vi "Calibration.vi"(6 "SN":T1, 7 "Show Front Panel":bool=TRUE, 8 "error in (no error)":errorcluster, 9 "file path (dialog if empty)":path=path "C:/Program Files/GE/Dryer Performance Test/CalibrationDates.txt", 10 "Calibration\nDue Date":T3 {"Chamber Temp" format="%<%x>T"; "Probe 2 Temp" format="%<%x>T"; "Probe 1 Temp" format="%<%x>T"; "TC Panel 2" format="%<%x>T"; "TC Panel 1" format="%<%x>T"; "NI DAQ Card 7" format="%<%x>T"; "NI DAQ Card 6" format="%<%x>T"; "NI DAQ Card 5" format="%<%x>T"; "NI DAQ Card 4" format="%<%x>T"; "NI DAQ Card 3" format="%<%x>T"; "NI DAQ Card 2" format="%<%x>T"; "NI DAQ Card 1" format="%<%x>T"; "Gas Meter Thermocouple" format="%<%x>T"; "Gas Meter Pressure Transducer" format="%<%x>T"; "Gas Meter" format="%<%x>T"; "Sentra Scale" format="%<%x>T"; "B-Tech Scale" format="%<%x>T"; "Barometer" format="%<%x>T"; "WT 500" format="%<%x>T"; "Chroma" format="%<%x>T"}, 11 "Calibration ID":T2) -> (0 "error out":errorcluster, 4 "OutputData":string[][](array[string]))   [LabVIEW 2012]
uses:
  Calibration.ctl
  CalibrationTime.ctl
  Calibration_SN.ctl
  <vilib>/Utility/file.llb/Write To Spreadsheet File (string).vi
panel:
  in  "Size":i32
  out "snta":string[](array[string])
  in  "Tab Control":enum32{"Calibration Dates", "File Location"}(tab)
  in  "Complete":bool
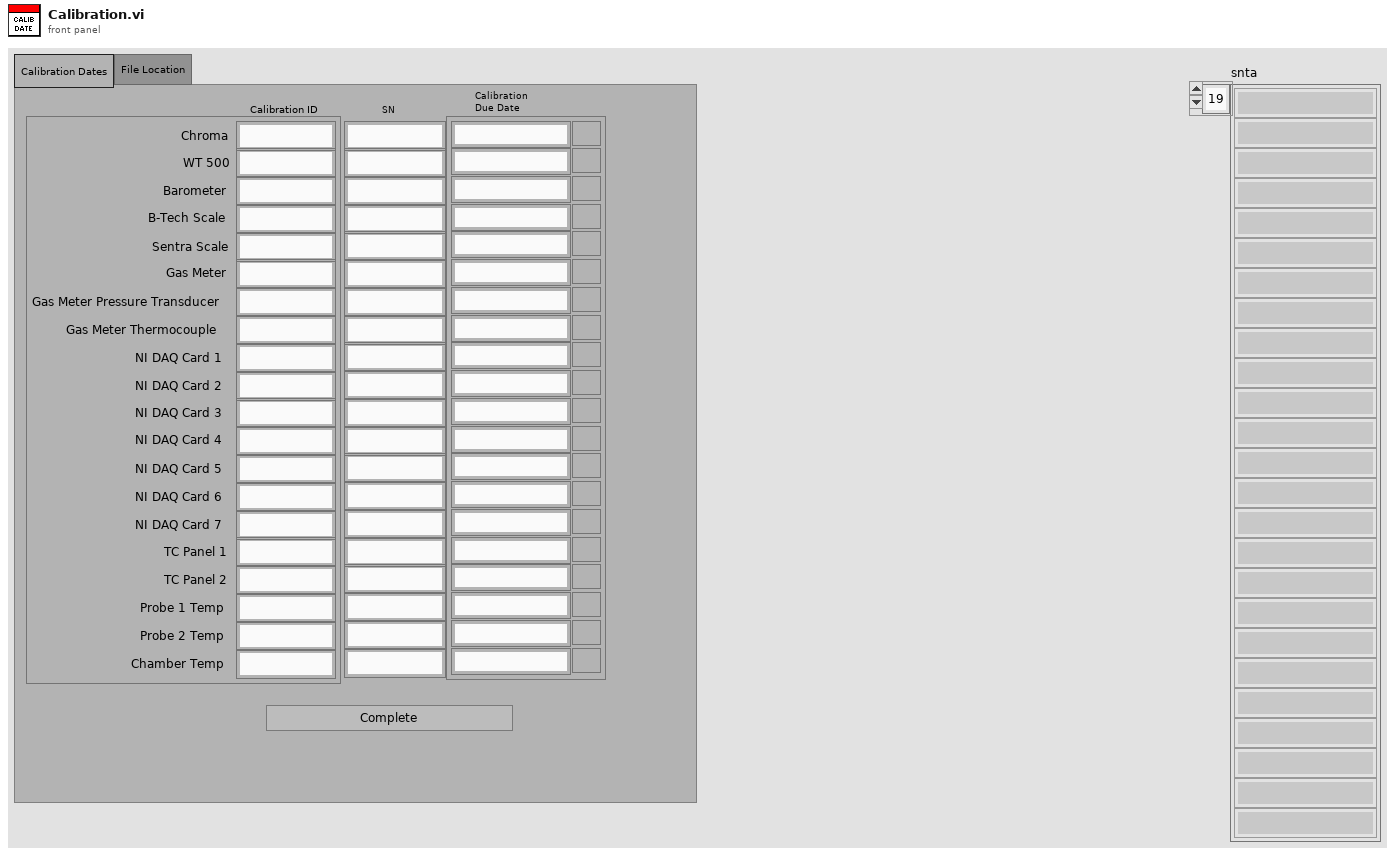
[diagram p1: front panel]
types:
  T1 = typedef "Calibration_SN.ctl" = cluster{"Chroma":string, "WT 500":string, "Barometer":string, "B-Tech Scale":string, "Sentra Scale":string, "Gas Meter":string, "Gas Meter Pressure Transducer":string, "Gas Meter Thermocouple":string, "NI DAQ Card 1":string, "NI DAQ Card 2":string, "NI DAQ Card 3":string, "NI DAQ Card 4":string, "NI DAQ Card 5":string, "NI DAQ Card 6":string, "NI DAQ Card 7":string, "TC Panel 1":string, "TC Panel 2":string, "Probe 1 Temp":string, "Probe 2 Temp":string, "Chamber Temp":string}
  T2 = typedef "Calibration.ctl" = cluster{"Chroma":string, "WT 500":string, "Barometer":string, "B-Tech Scale":string, "Sentra Scale":string, "Gas Meter":string, "Gas Meter Pressure Transducer":string, "Gas Meter Thermocouple":string, "NI DAQ Card 1":string, "NI DAQ Card 2":string, "NI DAQ Card 3":string, "NI DAQ Card 4":string, "NI DAQ Card 5":string, "NI DAQ Card 6":string, "NI DAQ Card 7":string, "TC Panel 1":string, "TC Panel 2":string, "Probe 1 Temp":string, "Probe 2 Temp":string, "Chamber Temp":string}
  T3 = typedef "CalibrationTime.ctl" = cluster{"Chroma":timestamp, "WT 500":timestamp, "Barometer":timestamp, "B-Tech Scale":timestamp, "Sentra Scale":timestamp, "Gas Meter":timestamp, "Gas Meter Pressure Transducer":timestamp, "Gas Meter Thermocouple":timestamp, "NI DAQ Card 1":timestamp, "NI DAQ Card 2":timestamp, "NI DAQ Card 3":timestamp, "NI DAQ Card 4":timestamp, "NI DAQ Card 5":timestamp, "NI DAQ Card 6":timestamp, "NI DAQ Card 7":timestamp, "TC Panel 1":timestamp, "TC Panel 2":timestamp, "Probe 1 Temp":timestamp, "Probe 2 Temp":timestamp, "Chamber Temp":timestamp}
  T4 = enum32{"invalid app kind", "Development System", "Run Time System", "Student Edition", "Embedded LabVIEW", "Evaluation", "Custom"}
  T5 = enum32{"Invalid", "Standard", "Closed", "Hidden", "Minimized", "Maximized"}
  T6 = cluster{"Core":cluster{"Current VI Reference":refnum<vi>, "Close Panel on Exit?":bool}, "Calibration\nDue Date":T3, "file path (dialog if empty)":path, "SN":T1, "Calibration ID":T2, "Total Array":string[][], "Size":i32}
  T7 = cluster{"Current VI Reference":refnum<vi>, "Close Panel on Exit?":bool}
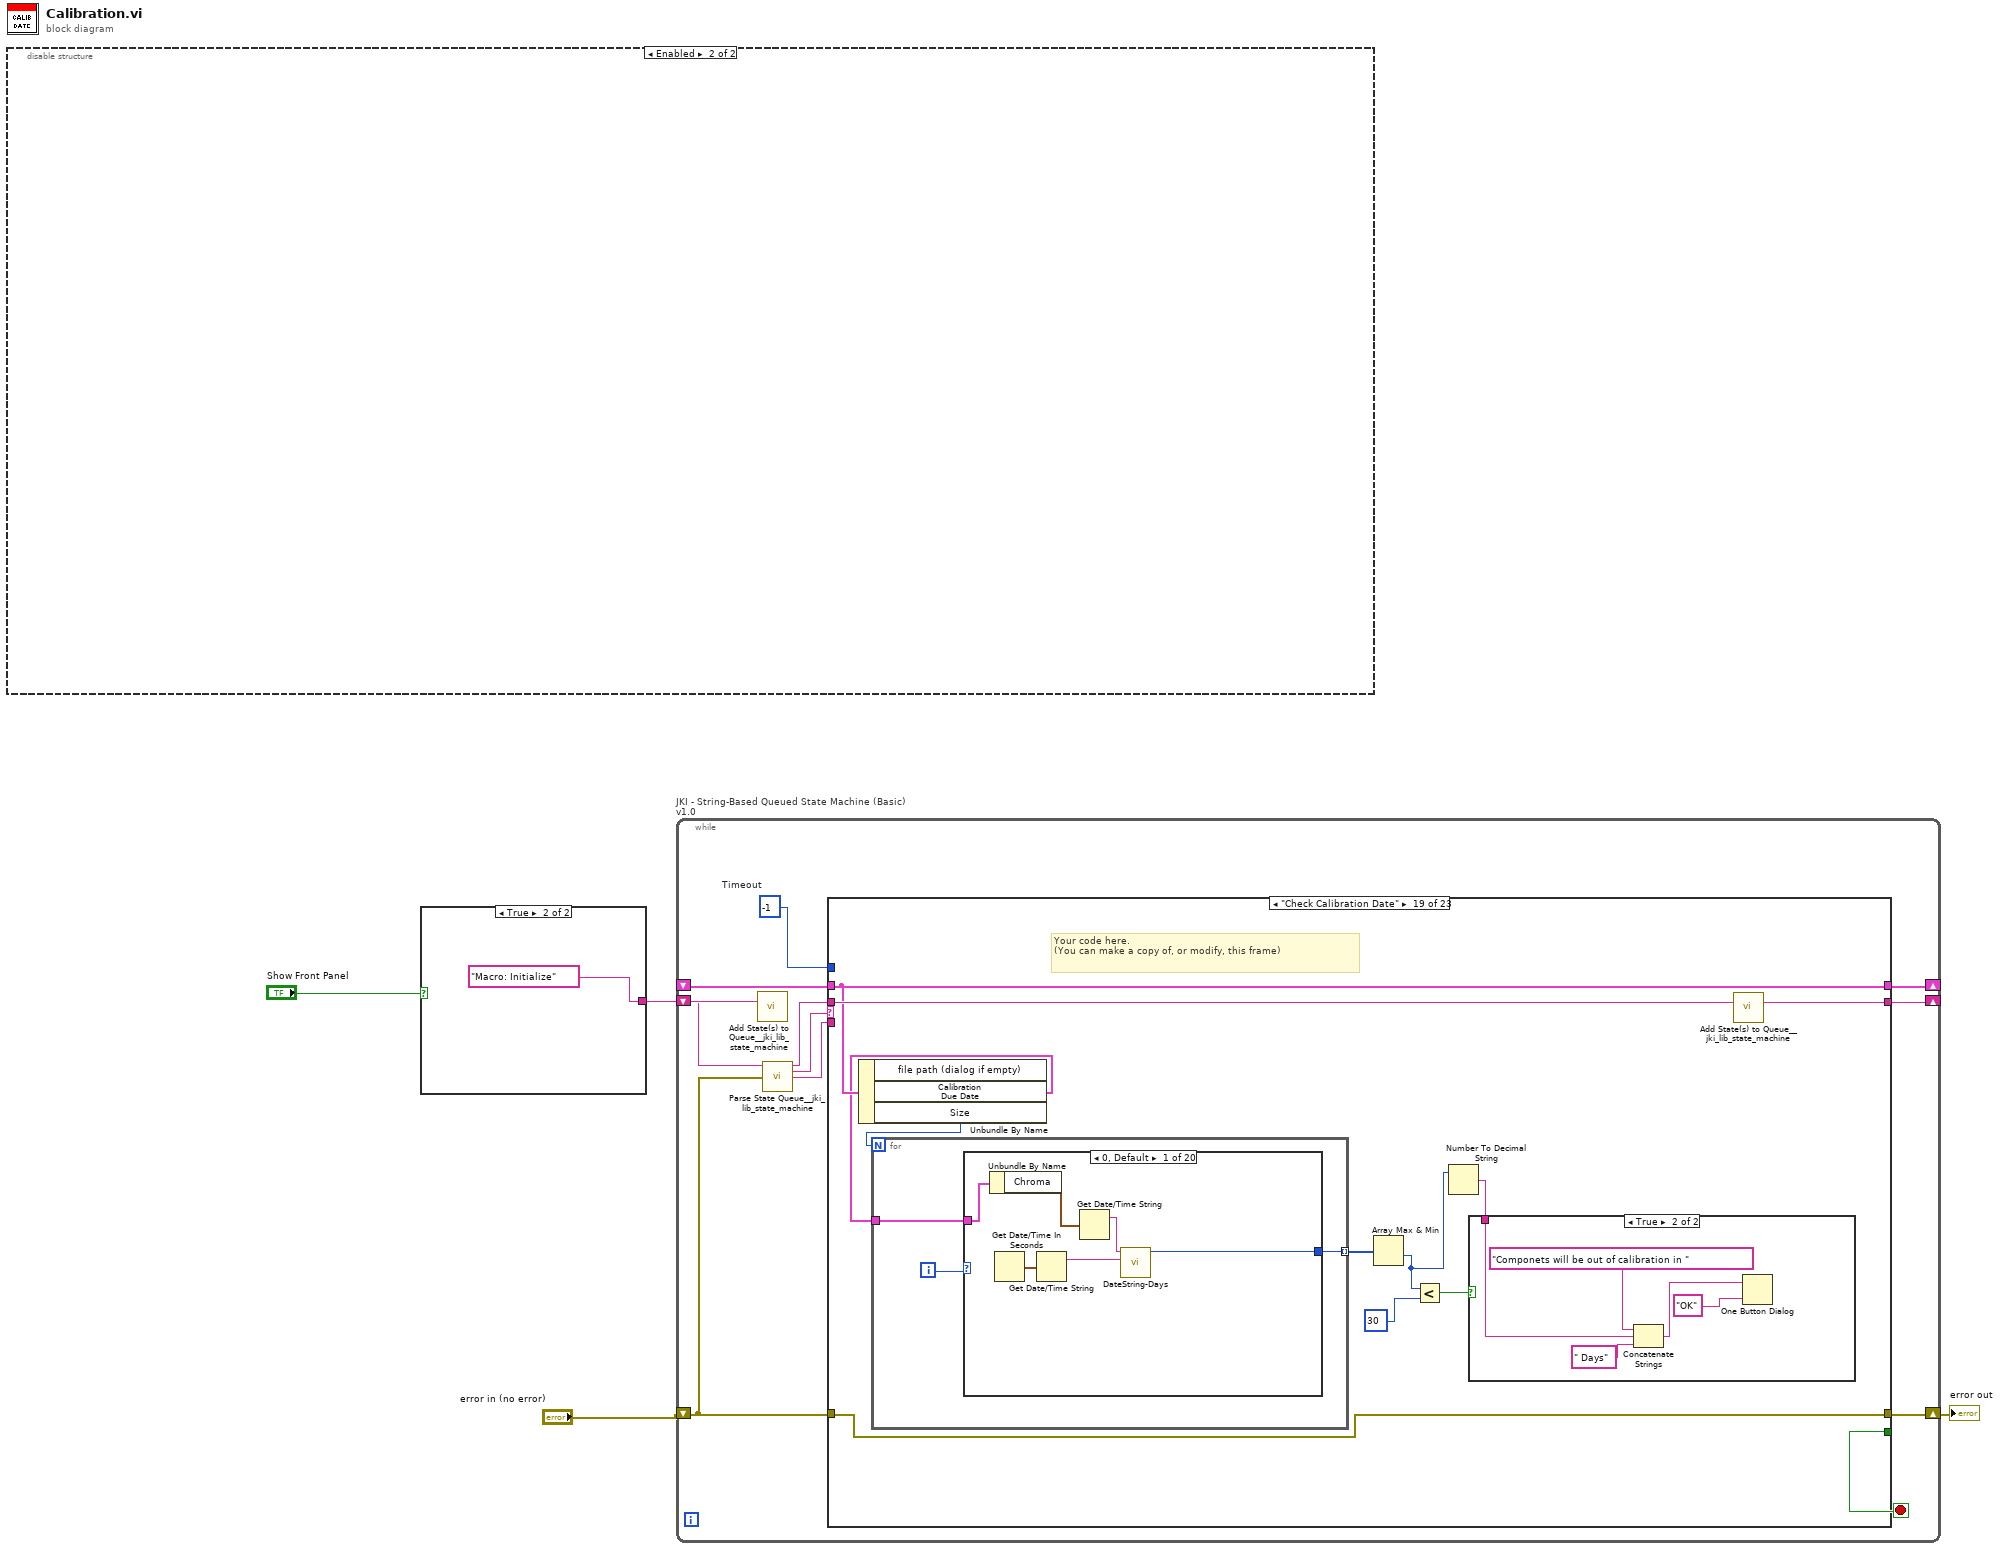
[diagram p0: block diagram]
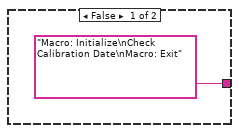
[diagram p2: hidden frame]
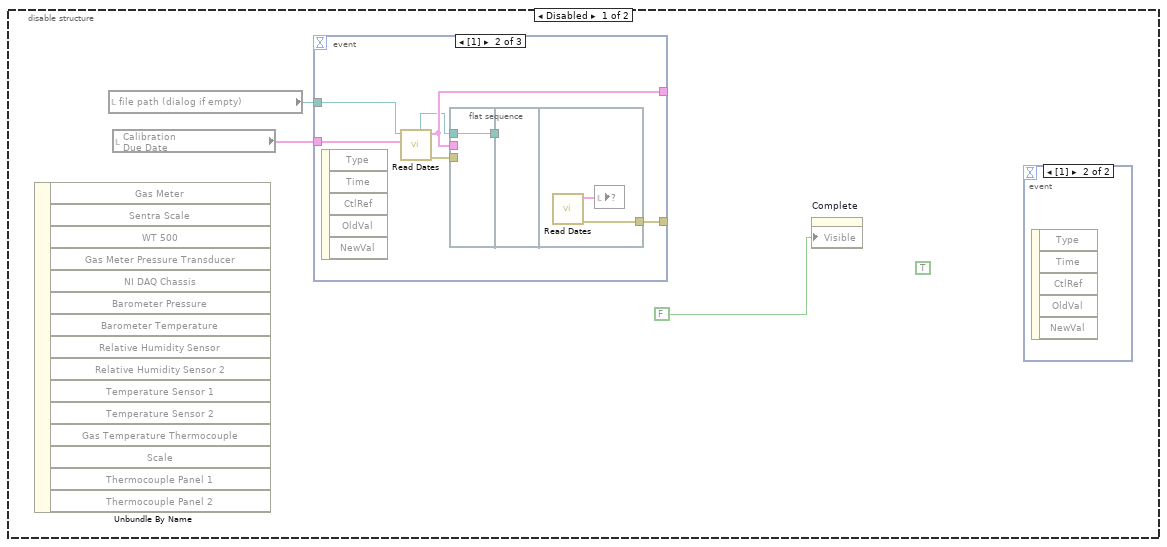
[diagram p3: hidden frame]
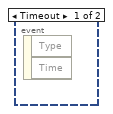
[diagram p4: hidden frame]
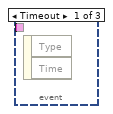
[diagram p5: hidden frame]
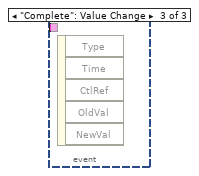
[diagram p6: hidden frame]
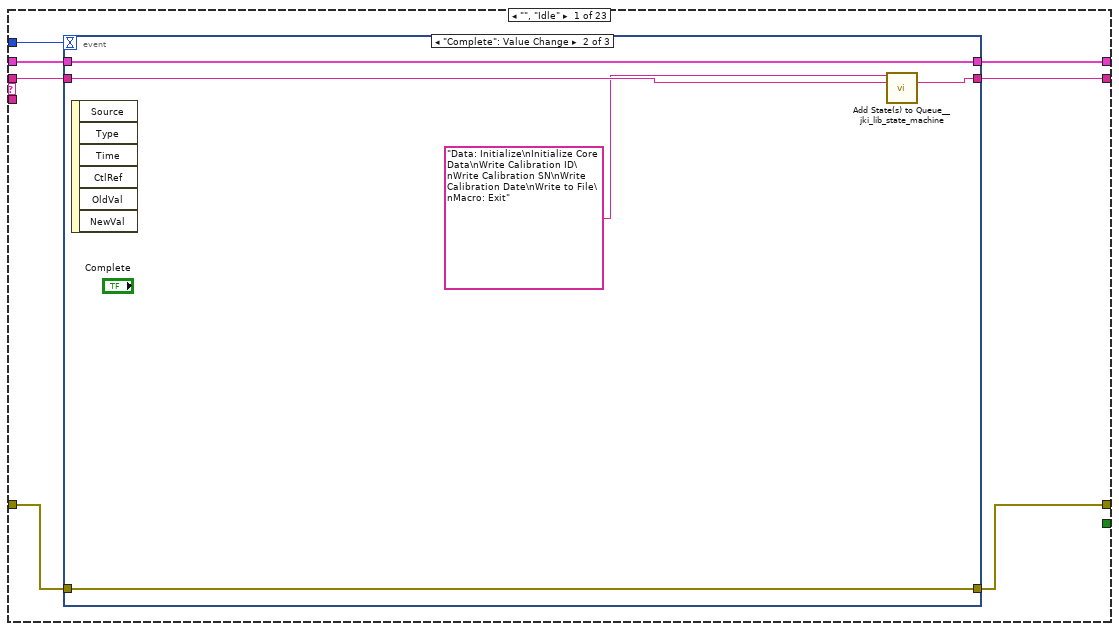
[diagram p7: hidden frame]
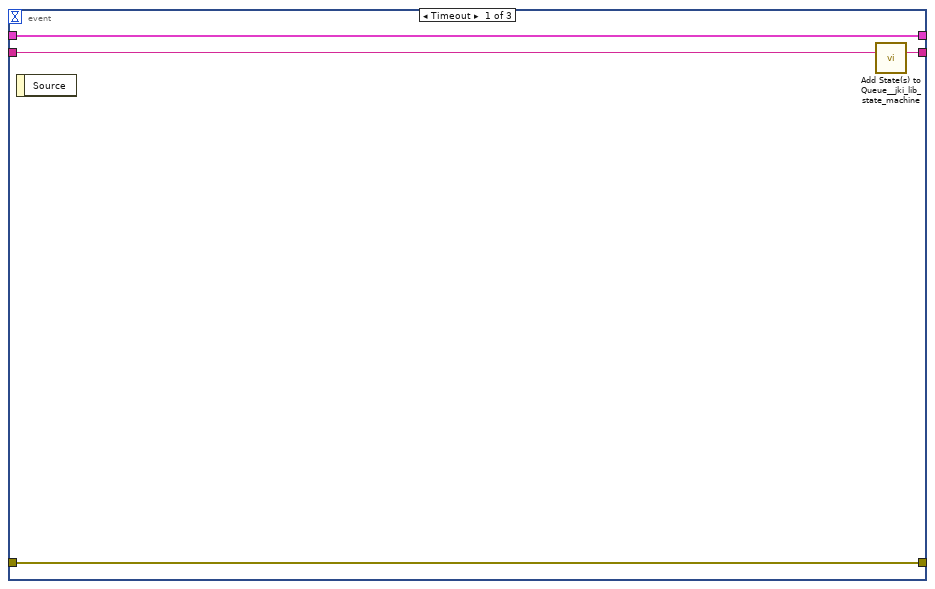
[diagram p8: hidden frame]
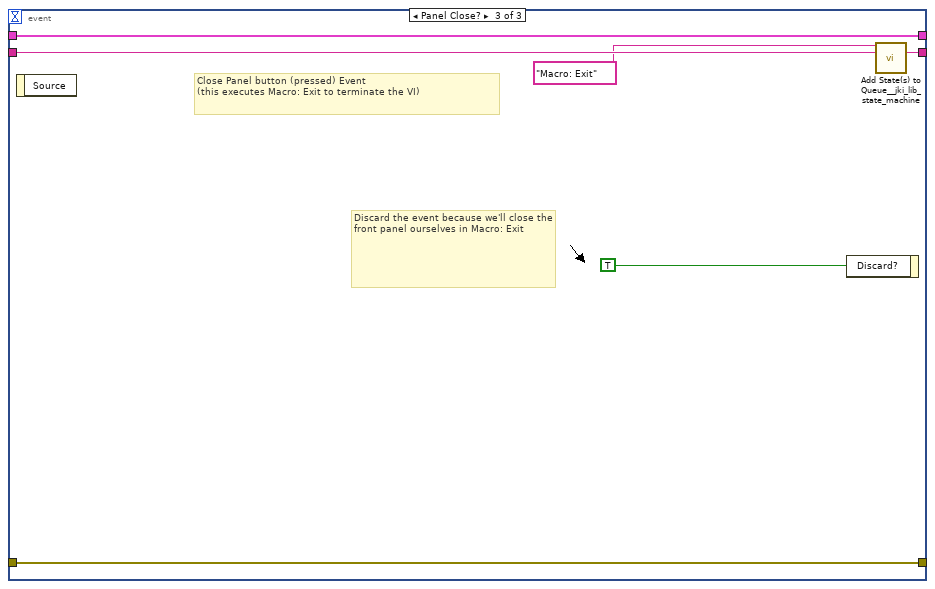
[diagram p9: hidden frame]
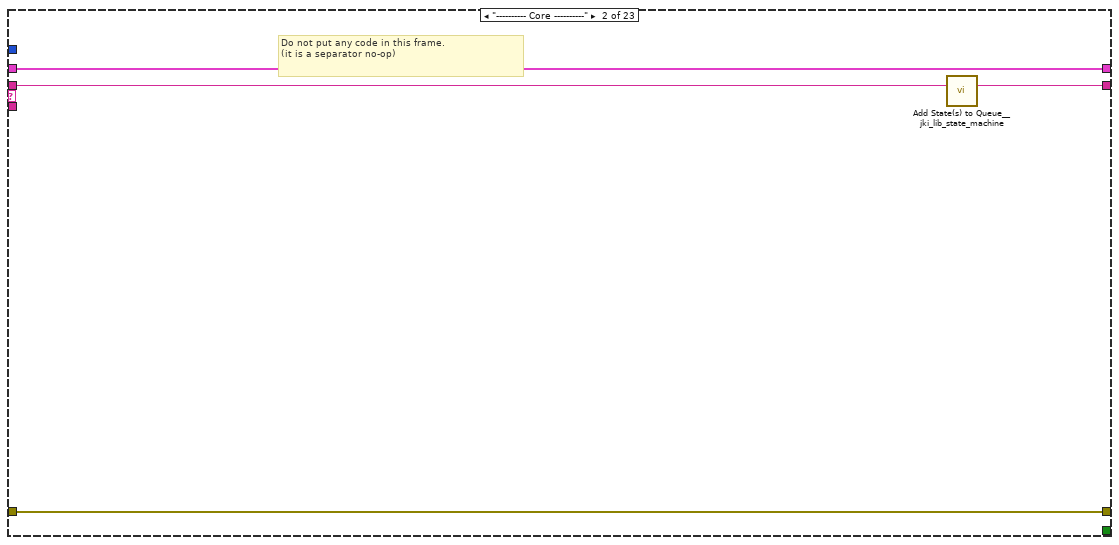
[diagram p10: hidden frame]
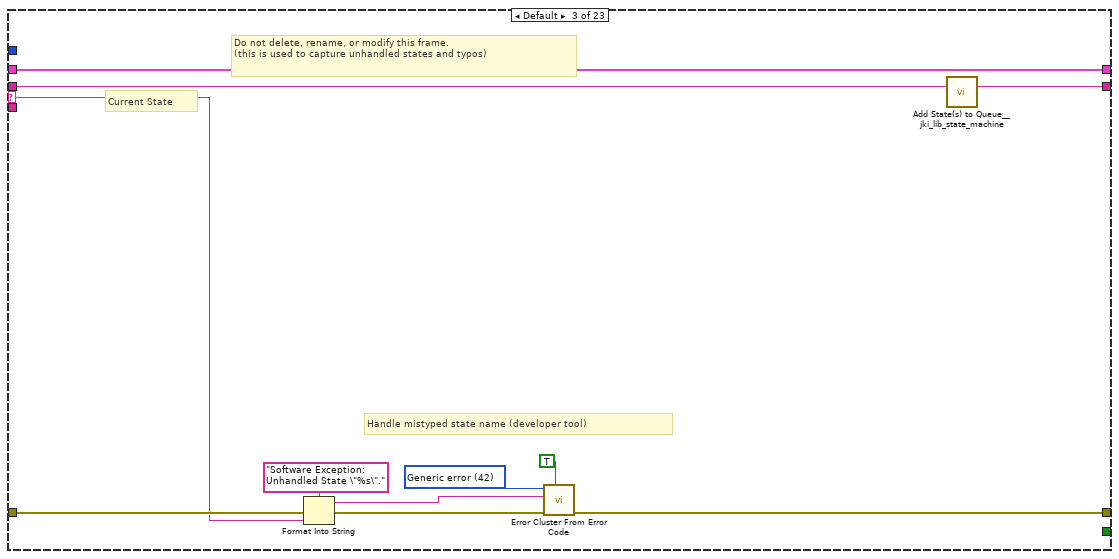
[diagram p11: hidden frame]
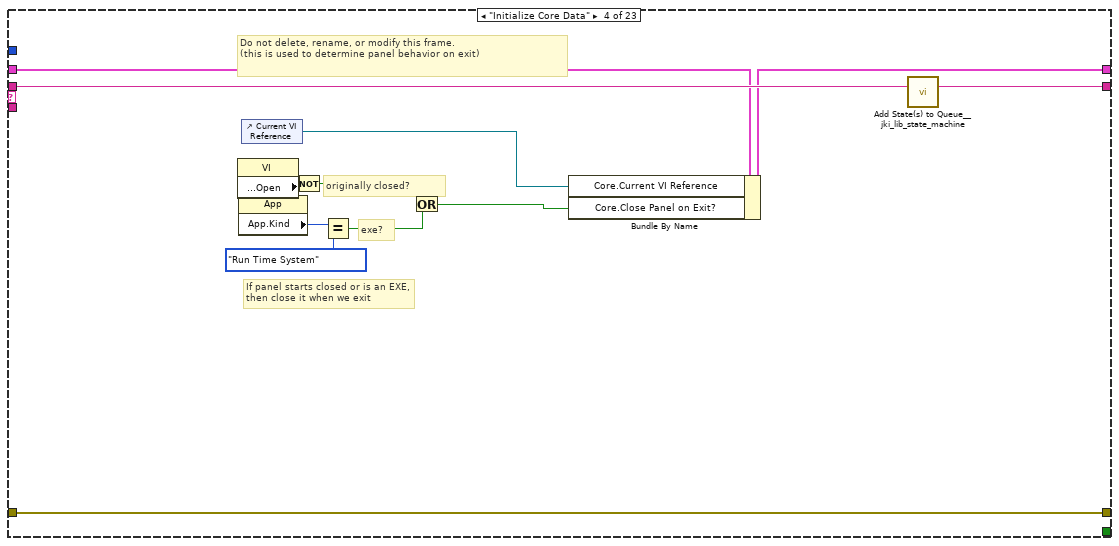
[diagram p12: hidden frame]
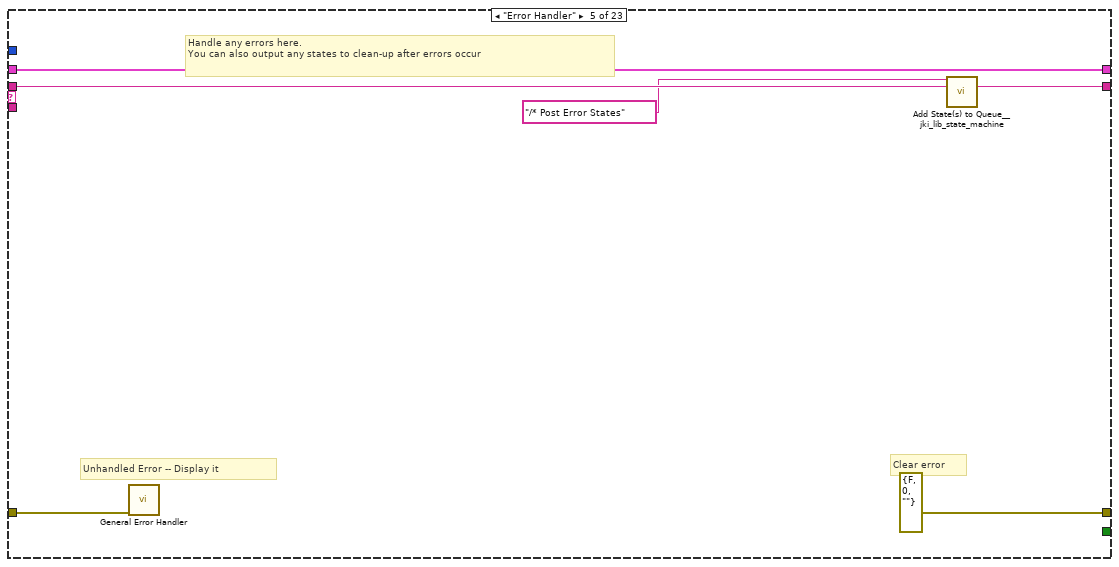
[diagram p13: hidden frame]
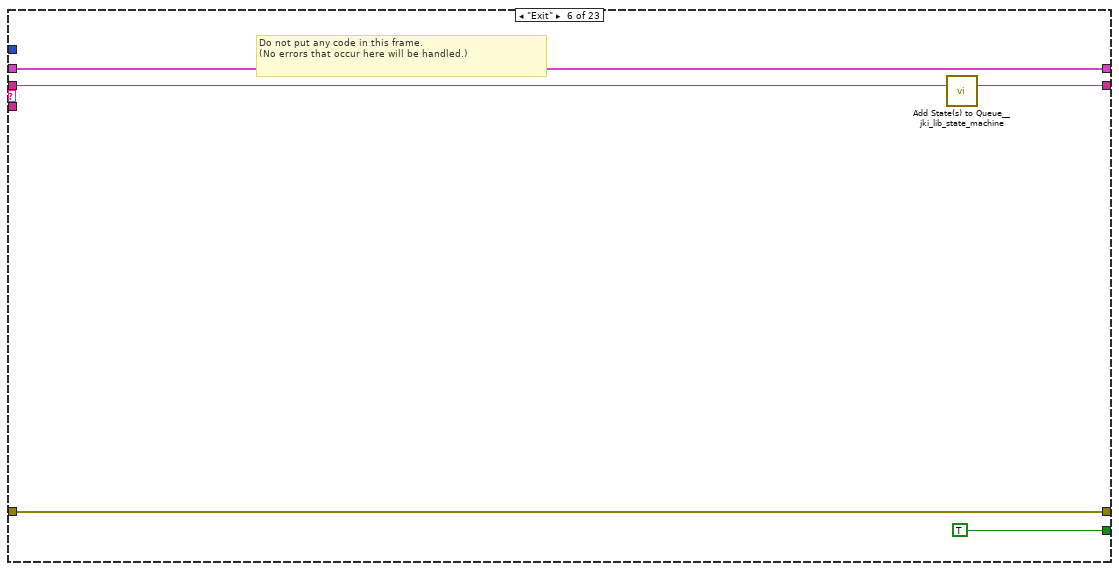
[diagram p14: hidden frame]
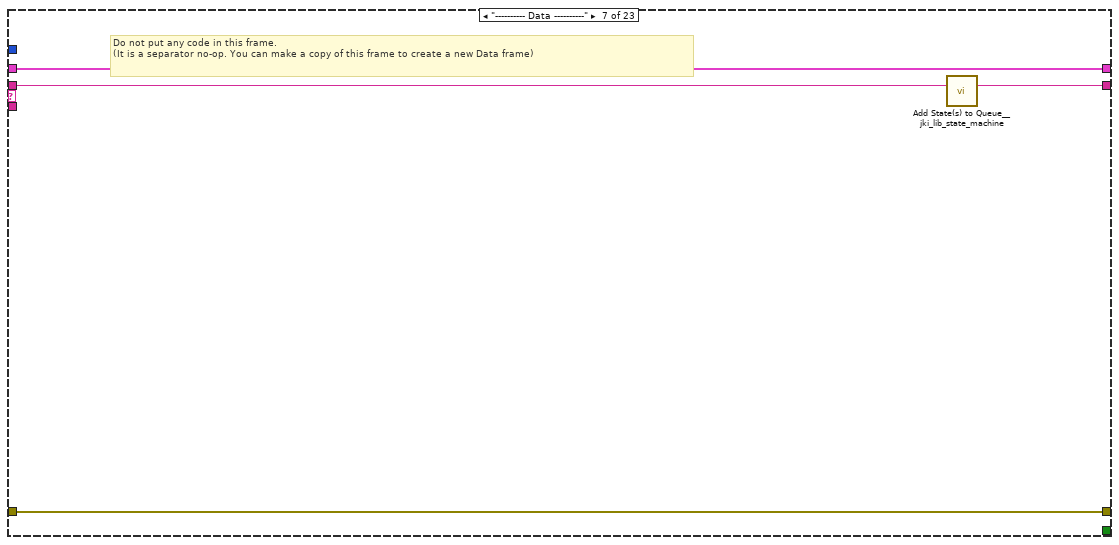
[diagram p15: hidden frame]
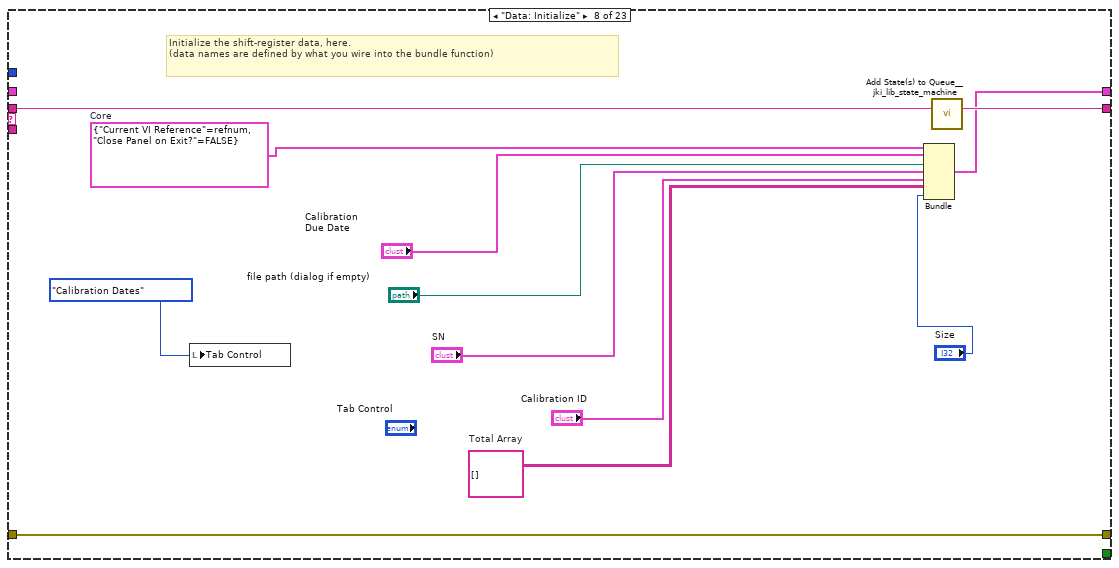
[diagram p16: hidden frame]
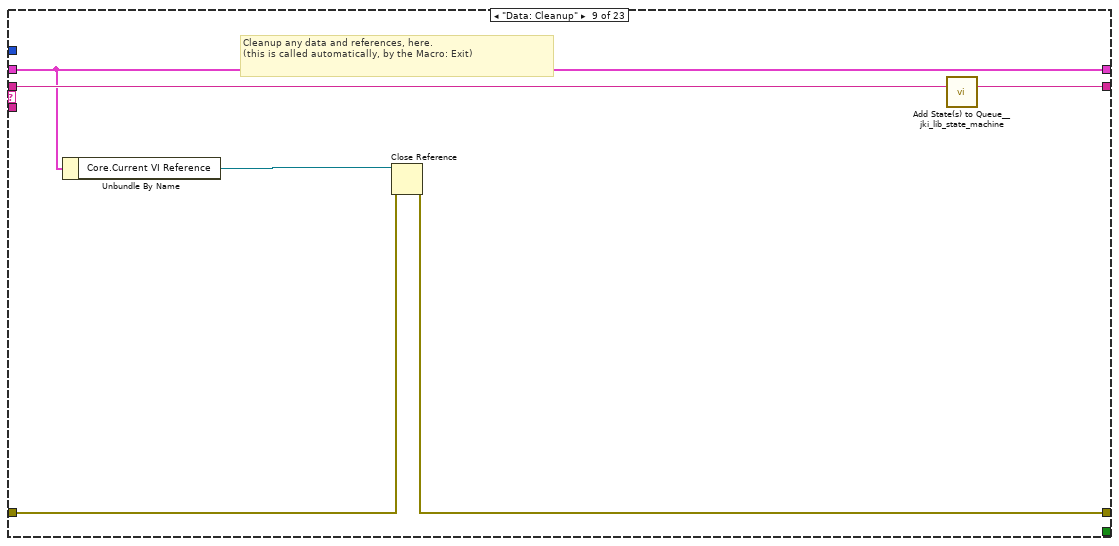
[diagram p17: hidden frame]
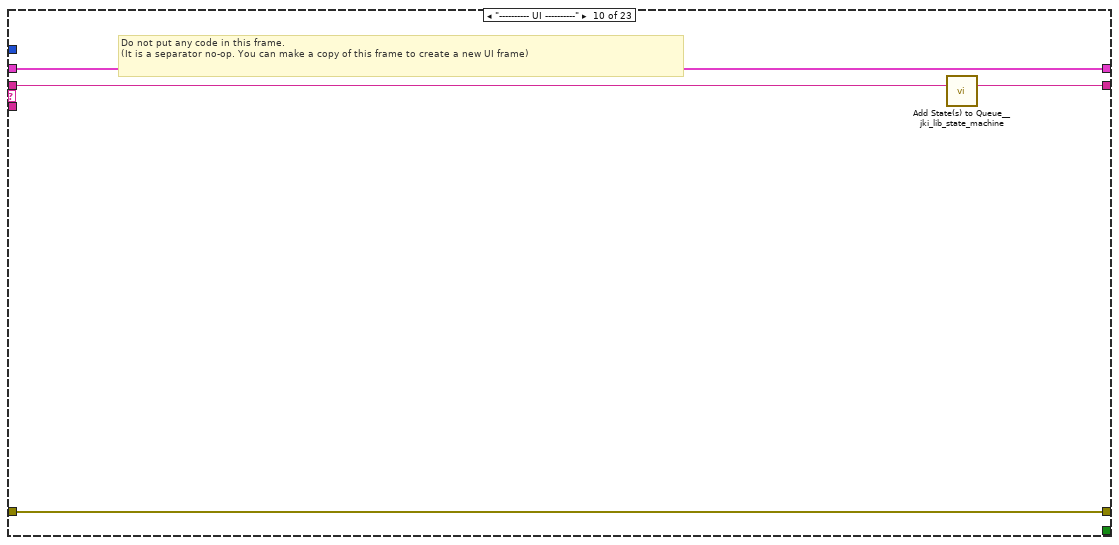
[diagram p18: hidden frame]
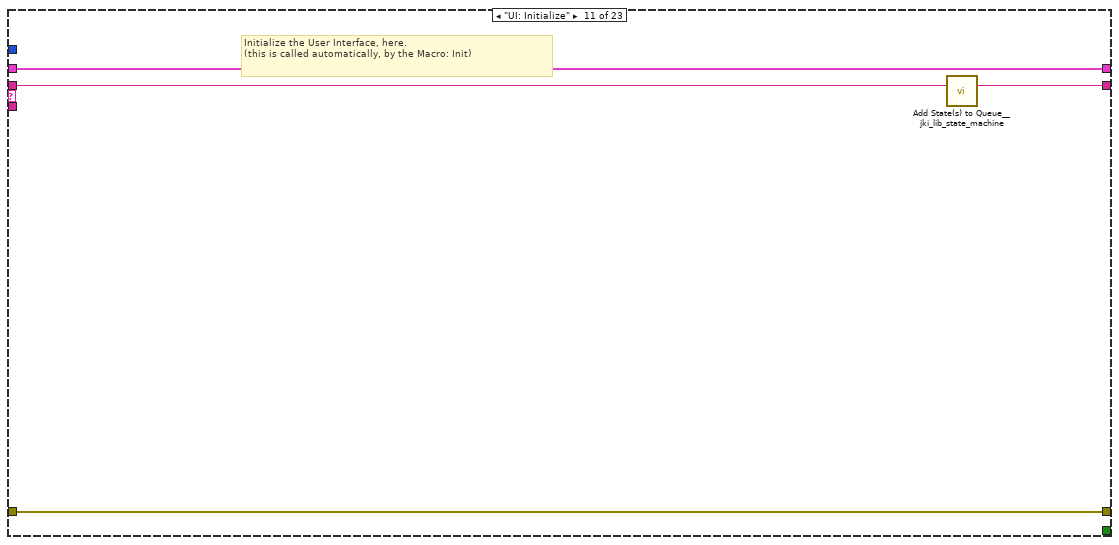
[diagram p19: hidden frame]
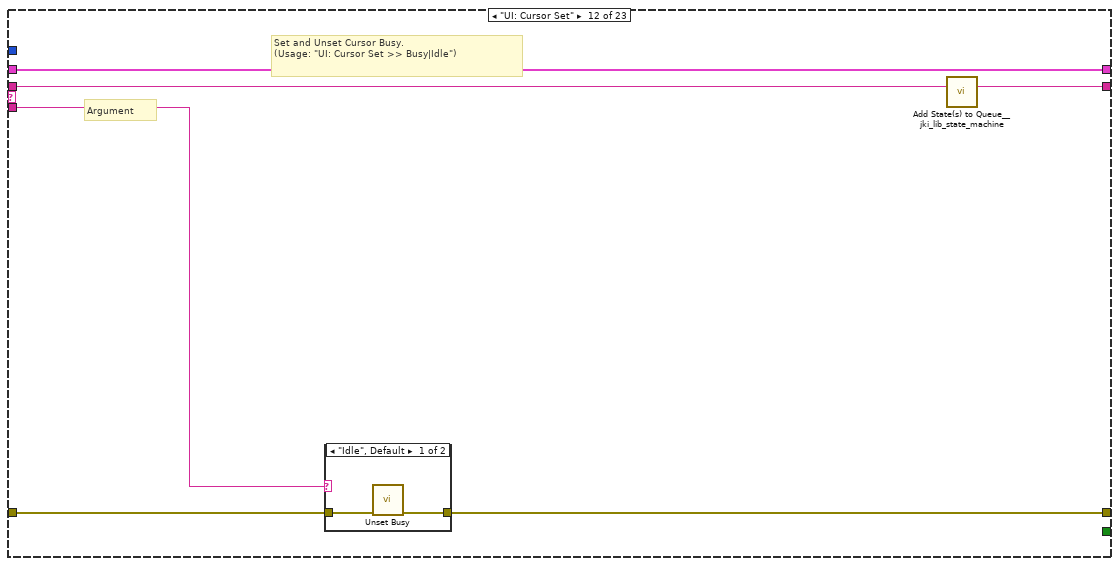
[diagram p20: hidden frame]
diagram:
  n1 = disable-structure shown="Enabled" {
    frame Disabled {
      w8 = TRUE ("Visible")
      n2 = Unbundle By Name() -> ()  [unwired: 1 in, 15 out]
      n3 = local read "file path (dialog if empty)"() -> (w6:path)
      n4 = local read "Calibration\nDue Date"() -> (w7:T3)
      n5 = event shown="[1]" {
        selector: _ -> [_ _ _]
        dyn-events: _ -> [_ _ _]
        timeout: _ -> [_ _ _]
        tunnel: [_ w13 _] -> _
        tunnel: [_ w17 _] -> _
        tunnel: w7 -> [_ w15 _]
        tunnel: w6 -> [_ w14 _]
        event Timeout {
          n6 = event-data() -> ()  [unwired: 1 in, 2 out]
        }
        event #1 (no event record) {
          n7 = event-data() -> ()  [unwired: 1 in, 5 out]
          n8 = call "Read Dates.vi"("Time Stamp in"=w15, "file path (dialog if empty)"=w14) -> ("error out"=w12:errorcluster, "Time Stamp out"=w13:T3, "new file path (Not A Path if cancelled)"=w11:path)  [unwired: 4 in, 3 out]
          n9 = flat-sequence {
            tunnel: w12 -> [_]
            tunnel: w11 -> [w18]
            tunnel: w13 -> [_]
            tunnel: [w18] -> w16
            tunnel: w16 -> [_]
            tunnel: [w19] -> w17
            frame #0 {
            }
            frame #1 {
            }
            frame #2 {
              n10 = call "Read Dates.vi"() -> ("error out"=w19:errorcluster, "Time Stamp out"=w20:T3)  [unwired: 6 in, 4 out]
              n11 = local write item#-1(w20) -> ()
            }
          }
        }
        event "Complete": Value Change {
          n12 = event-data() -> ()  [unwired: 1 in, 5 out]
        }
      }
      n13 = property on="Complete" class="Bool"("Visible"=FALSE) -> (error out=w9:errorcluster)  [unwired: 2 in, 1 out]
      n14 = event shown="[1]" {
        selector: _ -> [_ _]
        dyn-events: _ -> [_ _]
        timeout: _ -> [_ _]
        event Timeout {
          n15 = event-data() -> ()  [unwired: 1 in, 2 out]
        }
        event #1 (no event record) {
          n16 = event-data() -> ()  [unwired: 1 in, 5 out]
        }
      }
    }
    frame Enabled {
    }
  }
  n17 = case shown="True" "Show Front Panel" {
    tunnel: ["Macro: Initialize\nCheck Calibration Date\nMacro: Exit" "Macro: Initialize"] -> w4
    frame False {
    }
    frame True {
    }
  }
  n18 = call <vilib>:"Add State(s) to Queue__jki_lib_state_machine.vi"("State(s) in (\"\")"=w4) -> ("States Out"=w5:string)  [unwired: 14 in]
  n19 = while "JKI - String-Based Queued State Machine (Basic) v1.0" {
    shift-right: [w26] -> _
    shift-left: _ -> [w25]
    shift-right: [w29] -> w2
    shift-left: "error in (no error)" -> [w23]
    shift-right: [w28] -> _
    shift-left: w5 -> [w30]
    stop <- w27 stop-if-true
    w24 = -1  # Timeout
    n20 = call <vilib>:"Parse State Queue__jki_lib_state_machine.vi"("State Queue"=w30, "Error In (no error)"=w23) -> ("Remaining States"=w32:string, "Current State"=w33:string, "Arguments"=w31:string)  [unwired: 11 in]
    n21 = case shown="\"Check Calibration Date\"" w33 {
      selector: w33 -> [_ _ w60 _ _ _ _ _ _ _ _ _ _ _ _ _ _ _ _ _ _ _ _]
      tunnel: w32 -> [w40 w59 w64 w82 w88 w93 w97 w109 w115 w119 w123 w129 w140 w166 w171 w181 w185 w202 w213 w355 w433 w447 w507]
      tunnel: w31 -> [_ _ _ _ _ _ _ _ _ _ _ w124 w134 _ _ _ _ _ _ _ _ _ _]
      tunnel: w25 -> [w38 w56 w62 w73 w85 w91 w94 _ w110 w116 w121 w127 w136 w163 w168 w178 w182 w198 w211 w348 w431 w441 w501]
      tunnel: [w37 w57 w66 w79 errorcluster {"status"=FALSE, "code"=0, "source"=""} ("error out") w90 w95 w106 w111 w117 w120 w125 w137 w164 w169 w179 w183 w192 w210 w350 w428 w442 w502] -> w29
      tunnel: w23 -> [w36 w57 w65 w79 w84 w90 w95 w106 w112 w117 w120 w126 w138 w164 w169 w179 w183 w193 w210 w351 w428 w443 w503]
      tunnel: [w39 w58 w63 w81 w87 w92 w96 w108 w114 w118 w122 w128 w139 w165 w170 w180 w184 w201 w212 w354 w432 w446 w506] -> w28
      tunnel: [_ _ _ _ _ TRUE _ _ _ _ _ _ _ _ _ _ _ _ _ _ _ _ _] -> w27
      tunnel: [w35 w56 w62 w80 w85 w91 w94 w107 w110 w116 w121 w127 w136 w163 w168 w178 w182 w196 w211 w347 w431 w440 w500] -> w26
      tunnel: w24 -> [w34 _ _ _ _ _ _ _ _ _ _ _ _ _ _ _ _ _ _ _ _ _ _]
      frame "", "Idle" {
        n22 = event shown="[1] \"Complete\": Value Change" {
          selector: _ -> [_ _ _]
          dyn-events: _ -> [_ _ _]
          timeout: w34 -> [_ _ _]
          tunnel: w40 -> [w44 w48 w55]
          tunnel: [w43 w49 w54] -> w39
          tunnel: w38 -> [w41 w45 w52]
          tunnel: [w42 w47 w53] -> w37
          tunnel: w36 -> [w42 w47 w53]
          tunnel: [w41 w45 w52] -> w35
          event Timeout {
            n23 = event-data() -> ()  [unwired: 1 in, 1 out]
            n24 = call <vilib>:"Add State(s) to Queue__jki_lib_state_machine.vi"("State(s) in (\"\")"=w44) -> ("States Out"=w43:string)  [unwired: 14 in]
          }
          event "Complete": Value Change {
            n25 = event-data() -> ()  [unwired: 1 in, 6 out]
            n26 = call <vilib>:"Add State(s) to Queue__jki_lib_state_machine.vi"("State(s) in Front (\"\")"="Data: Initialize\nInitialize Core Data\nWrite Calibration ID\nWrite Calibration SN\nWrite Calibration Date\nWrite to File\nMacro: Exit", "State(s) in (\"\")"=w48) -> ("States Out"=w49:string)  [unwired: 13 in]
          }
          event Panel Close? {
            # "Discard the event because we'll close the front panel ourselves in Macro: Exit"
            # "Close Panel button (pressed) Event\n(this executes Macro: Exit to terminate the VI)"
            n27 = event-data() -> ()  [unwired: 1 in, 1 out]
            n28 = event-data("Discard?"=TRUE) -> ()  [unwired: 1 in, 1 out]
            n29 = call <vilib>:"Add State(s) to Queue__jki_lib_state_machine.vi"("State(s) in Front (\"\")"="Macro: Exit", "State(s) in (\"\")"=w55) -> ("States Out"=w54:string)  [unwired: 13 in]
          }
        }
      }
      frame "---------- Core ----------" {
        # "Do not put any code in this frame.\n(it is a separator no-op)"
        n30 = call <vilib>:"Add State(s) to Queue__jki_lib_state_machine.vi"("State(s) in (\"\")"=w59) -> ("States Out"=w58:string)  [unwired: 14 in]
      }
      frame Default {
        w69 = 42 items=["No error", "Argument error", "Memory is full", "Out of zone", "End of file", "File already open", "Generic file I/O error", "File not found", "File permission error", "Disk is full", "Duplicate path", "Too many files open", "System feature not enabled", "Resource file not found", "Cannot add resource", "Resource not found", "Image not found", "Image memory error", "Pen does not exist", "Config type invalid", "Config token not found", "Config parse error", "Config memory error", "Bad external code format", "Bad external code offset", "External code not present", "Null window", "Destroy window error", "Null menu", "Print aborted", "Bad print record", "Print driver error", "Windows error during printing", "Memory error during printing", "Print dialog error", "Generic print error", "Invalid device refnum", "Device not found", "Device parameter error", "Device unit error", "Cannot open device", "Device call aborted", "Generic error", "Cancelled by user", "Object ID too low", "Object ID too high", "Object not in heap", "Unknown heap", "Unknown object (invalid DefProc)", "Unknown object (DefProc not in table)", "Message out of range", "Invalid (null) method", "Unknown message", "Manager call not supported", "Bad address", "Network operation in progress", "Network operation timed out", "Connection is busy", "Network attribute not supported", "Network error", "Address in use", "System out of memory", "Connection aborted", "Connection refused", "Not connected", "Already connected", "Connection closed", "Initialization error (interapplication manager)", "Bad occurrence", "Wait on unbound occurrence handler", "Occurrence queue overflow", "Datalog type conflict", "Unused", "Unrecognized type (interapplication manager)", "Memory corrupt", "Failed to make temporary DLL", "Old CIN version", "Drag socket not found", "Failed to load drop-object", "Failed to register OLE object", "Failed to release OLE object", "Format specifier type mismatch", "Unknown format specifier", "Too few format specifiers", "Too many format specifiers", "Scan failed", "Newer CIN version", "Error converting to variant", "Runtime menu error", "Password tampered", "Variant attribute not found", "Incompatible variant data type", "Event data is not available", "Event Store is not present", "Occurrence is not found", "Event Queue is not created", "Event info is not available", "Refnum passed is NULL", "Error retrieving Class GUID", "Error retrieving CoClass GUID", "Error retrieving TypeLib GUID.", "Bad built application magic bytes.", "Specific driver is different from the specific driver associated with the Logical Name.", "There is no session opened to the class driver.", "Max Error", "MAX - Error with config objects", "MAX - Error loading configuration", "MAX - Group not supported"]
        # "Current State"
        # "Do not delete, rename, or modify this frame.\n(this is used to capture unhandled states and typos)"
        # "Handle mistyped state name (developer tool)"
        n31 = Format Into String(format string="Software Exception: Unhandled State \"%s\"." ("message"), error in=w65, w60) -> (resulting string=w68:string, error out=w67:errorcluster)  [unwired: 1 in]
        n32 = call <vilib>:"Error Cluster From Error Code.vi"("show call chain? (False)"=TRUE, "error in (no error)"=w67, "error message (\"\")"=w68, "error code (0)"=w69) -> ("error out"=w66:errorcluster)  [unwired: 5 in]
        n33 = call <vilib>:"Add State(s) to Queue__jki_lib_state_machine.vi"("State(s) in (\"\")"=w64) -> ("States Out"=w63:string)  [unwired: 14 in]
      }
      frame "Initialize Core Data" {
        # "Do not delete, rename, or modify this frame.\n(this is used to determine panel behavior on exit)"
        # "originally closed?"
        # "exe?"
        # "If panel starts closed or is an EXE, then close it when we exit"
        n34 = property class="VI"() -> ("Front Panel.Open"=w78:bool)  [unwired: 2 in, 2 out]
        n35 = property class="App"() -> ("App.Kind"=w77:T4)  [unwired: 2 in, 2 out]
        n36 = control-ref of="Current VI Reference"() -> (w71:refnum<vi>)
        n37 = Not(x=w78) -> (.not. x?=w75:bool)
        n38 = Equal?(x=w77, y=T4."Run Time System" ("Application:Kind")) -> (x = y?=w74:bool)
        n39 = Or(x=w75, y=w74) -> (x .or. y?=w72:bool)
        n40 = Bundle By Name(cluster=w73, "Core.Current VI Reference"=w71, "Core.Close Panel on Exit?"=w72) -> (w80:T6)
        n41 = call <vilib>:"Add State(s) to Queue__jki_lib_state_machine.vi"("State(s) in (\"\")"=w82) -> ("States Out"=w81:string)  [unwired: 14 in]
      }
      frame "Error Handler" {
        # "Unhandled Error -- Display it"
        # "Handle any errors here.\nYou can also output any states to clean-up after errors occur"
        # "Clear error"
        n42 = call <vilib>:"General Error Handler.vi"("error in (no error)"=w84) -> ()  [unwired: 10 in, 5 out]
        n43 = call <vilib>:"Add State(s) to Queue__jki_lib_state_machine.vi"("State(s) in Front (\"\")"="/* Post Error States", "State(s) in (\"\")"=w88) -> ("States Out"=w87:string)  [unwired: 13 in]
      }
      frame "Exit" {
        # "Do not put any code in this frame.\n(No errors that occur here will be handled.)"
        n44 = call <vilib>:"Add State(s) to Queue__jki_lib_state_machine.vi"("State(s) in (\"\")"=w93) -> ("States Out"=w92:string)  [unwired: 14 in]
      }
      frame "---------- Data ----------" {
        # "Do not put any code in this frame.\n(It is a separator no-op. You can make a copy of this frame to create a new Data frame)"
        n45 = call <vilib>:"Add State(s) to Queue__jki_lib_state_machine.vi"("State(s) in (\"\")"=w97) -> ("States Out"=w96:string)  [unwired: 14 in]
      }
      frame "Data: Initialize" {
        w100 = string[][] []  # Total Array
        w105 = T7 {"Current VI Reference"=refnum, "Close Panel on Exit?"=FALSE}  # Core
        # "Initialize the shift-register data, here.\n(data names are defined by what you wire into the bundle function)"
        n46 = local write "Tab Control"(enum32{"Calibration Dates", "File Location"}."Calibration Dates" ("Tab Control")) -> ()
        n47 = Bundle("Core"=w105, "Calibration\nDue Date"="Calibration\nDue Date", "file path (dialog if empty)"="file path (dialog if empty)", "SN"="SN", "Calibration ID"="Calibration ID", "Total Array"=w100, "Size"="Size") -> (w107:T6)  [unwired: 1 in]
        n48 = call <vilib>:"Add State(s) to Queue__jki_lib_state_machine.vi"("State(s) in (\"\")"=w109) -> ("States Out"=w108:string)  [unwired: 14 in]
      }
      frame "Data: Cleanup" {
        # "Cleanup any data and references, here.\n(this is called automatically, by the Macro: Exit)"
        n49 = Unbundle By Name(w110) -> ("Core.Current VI Reference"=w113:refnum<vi>)
        n50 = Close Reference(reference=w113, error in (no error)=w112) -> (error out=w111:errorcluster)
        n51 = call <vilib>:"Add State(s) to Queue__jki_lib_state_machine.vi"("State(s) in (\"\")"=w115) -> ("States Out"=w114:string)  [unwired: 14 in]
      }
      frame "---------- UI ----------" {
        # "Do not put any code in this frame.\n(It is a separator no-op. You can make a copy of this frame to create a new UI frame)"
        n52 = call <vilib>:"Add State(s) to Queue__jki_lib_state_machine.vi"("State(s) in (\"\")"=w119) -> ("States Out"=w118:string)  [unwired: 14 in]
      }
      frame "UI: Initialize" {
        # "Initialize the User Interface, here.\n(this is called automatically, by the Macro: Init)"
        n53 = call <vilib>:"Add State(s) to Queue__jki_lib_state_machine.vi"("State(s) in (\"\")"=w123) -> ("States Out"=w122:string)  [unwired: 14 in]
      }
      frame "UI: Cursor Set" {
        # "Argument"
        # "Set and Unset Cursor Busy.\n(Usage: \"UI: Cursor Set >> Busy|Idle\")"
        n54 = case shown="\"Idle\", Default" w124 {
          tunnel: w126 -> [w131 w133]
          tunnel: [w130 w132] -> w125
          frame "Idle", Default {
            n55 = call <vilib>:"Unset Busy.vi"("error in (no error)"=w131) -> ("error out"=w130:errorcluster)  [unwired: 10 in]
          }
          frame "Busy" {
            n56 = call <vilib>:"Set Busy.vi"("error in (no error)"=w133) -> ("error out"=w132:errorcluster)  [unwired: 9 in, 1 out]
          }
        }
        n57 = call <vilib>:"Add State(s) to Queue__jki_lib_state_machine.vi"("State(s) in (\"\")"=w129) -> ("States Out"=w128:string)  [unwired: 14 in]
      }
      frame "UI: Front Panel State" {
        # "Argument"
        # "Set Front Panel Open or Closed\n(Usage: \"UI: Front Panel State >> Open|Close\")"
        n58 = Unbundle By Name(w136) -> ("Core.Current VI Reference"=w135:refnum<vi>)
        n59 = case shown="\"Open\", Default" w134 {
          tunnel: w138 -> [w144 w157]
          tunnel: [w146 w158] -> w137
          tunnel: w135 -> [w145 w155]
          frame "Open", Default {
            n60 = property class="VI"(reference=w145, error in=w144) -> (reference out=w142:refnum<vi>, error out=w143:errorcluster, "Front Panel.Open"=w141:bool)
            n61 = case shown="True" w141 {
              tunnel: [w149 w152] -> w146
              tunnel: w143 -> [w148 w152]
              tunnel: w142 -> [w147 _]
              frame False {
                n62 = invoke class="VI" method="FP.Open"(reference=w147, error in=w148, "Activate"=TRUE, "State"=T5."Standard") -> (error out=w149:errorcluster)  [unwired: 1 in, 4 out]
              }
              frame True {
              }
            }
          }
          frame "Close" {
            n63 = property class="VI"(reference=w155, error in=w157) -> (reference out=w154:refnum<vi>, error out=w156:errorcluster, "Front Panel.Open"=w153:bool)
            n64 = case shown="True" w153 {
              tunnel: [w159 w162] -> w158
              tunnel: w156 -> [w159 w161]
              tunnel: w154 -> [_ w160]
              frame False {
              }
              frame True {
                n65 = invoke class="VI" method="FP.Close"(reference=w160, error in=w161) -> (error out=w162:errorcluster)  [unwired: 1 in, 2 out]
              }
            }
          }
        }
        n66 = call <vilib>:"Add State(s) to Queue__jki_lib_state_machine.vi"("State(s) in (\"\")"=w140) -> ("States Out"=w139:string)  [unwired: 14 in]
      }
      frame "---------- Macro ----------" {
        # "Do not put any code in this frame.\n(It is a separator no-op. You can make a copy of this frame to create a new Macro frame)"
        n67 = call <vilib>:"Add State(s) to Queue__jki_lib_state_machine.vi"("State(s) in (\"\")"=w166) -> ("States Out"=w165:string)  [unwired: 14 in]
      }
      frame "Macro: Initialize" {
        w167 = "Data: Initialize\nInitialize Core Data\nUI: Initialize\nUI: Front Panel State >> Open\nRead"  # Data: Initialize Initialize Core Data UI: Initialize UI: Front Panel State >> Open Read
        # "Initialization Macro\n(This is called once, when the VI starts)"
        n68 = call <vilib>:"Add State(s) to Queue__jki_lib_state_machine.vi"("State(s) in Front (\"\")"=w167, "State(s) in (\"\")"=w171) -> ("States Out"=w170:string)  [unwired: 13 in]
      }
      frame "Macro: Exit" {
        # "Exit Macro\n(This is called once, when the VI exits)"
        n69 = Unbundle By Name(w178) -> ("Core.Close Panel on Exit?"=w177:bool)
        n70 = Select(t="UI: Front Panel State >> Close", s=w177, f="") -> (s? t:f=w174:string)
        n71 = call <vilib>:"Add State(s) to Queue__jki_lib_state_machine.vi"("State(s) in (\"\")"=w174, "State(s) at Back (\"\")"="Data: Cleanup\nExit") -> ("States Out"=w172:string)  [unwired: 13 in]
        n72 = call <vilib>:"Add State(s) to Queue__jki_lib_state_machine.vi"("State(s) in Front (\"\")"=w172, "State(s) in (\"\")"=w181) -> ("States Out"=w180:string)  [unwired: 13 in]
      }
      frame "---------- New Category ----------" {
        # "Template Separator\n(You can make a copy of, or modify, this frame)"
        n73 = call <vilib>:"Add State(s) to Queue__jki_lib_state_machine.vi"("State(s) in (\"\")"=w185) -> ("States Out"=w184:string)  [unwired: 14 in]
      }
      frame "Read" {
        # "Your code here.\n(You can make a copy of, or modify, this frame)"
        n74 = Unbundle By Name(w198) -> ("file path (dialog if empty)"=w200:path, "Calibration\nDue Date"=w199:T3, "SN"=w194:T1, "Calibration ID"=w195:T2)
        n75 = call "Read Dates.vi"("SN"=w194, "error in (no error)"=w193, "Calibration ID"=w195, "Time Stamp in"=w199, "file path (dialog if empty)"=w200) -> ("error out"=w192:errorcluster, "SN."=w191:T1, "Calibration ID."=w190:T2, "Time Stamp out"=w197:T3, "Size"=w186:i32)  [unwired: 1 in, 1 out]
        n76 = Bundle By Name(cluster=w198, "Calibration\nDue Date"=w197, "SN"=w191, "Calibration ID"=w190, "Size"=w186) -> (w196:T6)
        n77 = Unbundle By Name(w196) -> ("Calibration\nDue Date"=w187:T3, "SN"=w188:T1, "Calibration ID"=w189:T2)
        n78 = property on="Calibration ID" class="Clust (strict)"("Value"=w189) -> ()  [unwired: 2 in, 2 out]
        n79 = property on="Calibration\nDue Date" class="Clust (strict)"("Value"=w187) -> ()  [unwired: 2 in, 2 out]
        n80 = call <vilib>:"Add State(s) to Queue__jki_lib_state_machine.vi"("State(s) in (\"\")"=w202) -> ("States Out"=w201:string)  [unwired: 14 in]
        n81 = property on="SN" class="Clust (strict)"("Value"=w188) -> ()  [unwired: 2 in, 2 out]
      }
      frame "Check Calibration Date" {
        # "Your code here.\n(You can make a copy of, or modify, this frame)"
        n82 = Unbundle By Name(w211) -> ("Calibration\nDue Date"=w209:T3, "Size"=w208:i32)  [unwired: 1 out]
        n83 = for {
          N: w208 -> [_]
          tunnel: w209 -> [w221]
          tunnel: [w219] -> w207 mode=indexing
          i -> [w220]
          n84 = case shown="0, Default" w220 {
            tunnel: w221 -> [w227 w233 w239 w245 w251 w257 w263 w269 w275 w281 w287 w293 w299 w305 w311 w317 w323 w329 w335 w341]
            tunnel: [w222 w228 w234 w240 w246 w252 w258 w264 w270 w276 w282 w288 w294 w300 w306 w312 w318 w324 w330 w336] -> w219
            frame 0, Default {
              n85 = Unbundle By Name(w227) -> ("Chroma"=w225:timestamp)
              n86 = Get Date/Time In Seconds() -> (seconds since 1Jan1904=w226:timestamp)
              n87 = Get Date/Time String(seconds (now)=w226) -> (date string=w223:string)  [unwired: 2 in, 1 out]
              n88 = Get Date/Time String(seconds (now)=w225) -> (date string=w224:string)  [unwired: 2 in, 1 out]
              n89 = call "DateString-Days.vi"("First date"=w223, "Second date"=w224) -> ("Elapsed days"=w222:i32)  [unwired: 8 in, 1 out]
            }
            frame 1 {
              n90 = Unbundle By Name(w233) -> ("WT 500"=w229:timestamp)
              n91 = Get Date/Time In Seconds() -> (seconds since 1Jan1904=w232:timestamp)
              n92 = Get Date/Time String(seconds (now)=w232) -> (date string=w230:string)  [unwired: 2 in, 1 out]
              n93 = Get Date/Time String(seconds (now)=w229) -> (date string=w231:string)  [unwired: 2 in, 1 out]
              n94 = call "DateString-Days.vi"("First date"=w230, "Second date"=w231) -> ("Elapsed days"=w228:i32)  [unwired: 8 in, 1 out]
            }
            frame 2 {
              n95 = Unbundle By Name(w239) -> ("Barometer"=w235:timestamp)
              n96 = Get Date/Time In Seconds() -> (seconds since 1Jan1904=w238:timestamp)
              n97 = Get Date/Time String(seconds (now)=w238) -> (date string=w236:string)  [unwired: 2 in, 1 out]
              n98 = Get Date/Time String(seconds (now)=w235) -> (date string=w237:string)  [unwired: 2 in, 1 out]
              n99 = call "DateString-Days.vi"("First date"=w236, "Second date"=w237) -> ("Elapsed days"=w234:i32)  [unwired: 8 in, 1 out]
            }
            frame 3 {
              n100 = Unbundle By Name(w245) -> ("B-Tech Scale"=w241:timestamp)
              n101 = Get Date/Time In Seconds() -> (seconds since 1Jan1904=w244:timestamp)
              n102 = Get Date/Time String(seconds (now)=w244) -> (date string=w242:string)  [unwired: 2 in, 1 out]
              n103 = Get Date/Time String(seconds (now)=w241) -> (date string=w243:string)  [unwired: 2 in, 1 out]
              n104 = call "DateString-Days.vi"("First date"=w242, "Second date"=w243) -> ("Elapsed days"=w240:i32)  [unwired: 8 in, 1 out]
            }
            frame 4 {
              n105 = Unbundle By Name(w251) -> ("Sentra Scale"=w247:timestamp)
              n106 = Get Date/Time In Seconds() -> (seconds since 1Jan1904=w250:timestamp)
              n107 = Get Date/Time String(seconds (now)=w250) -> (date string=w248:string)  [unwired: 2 in, 1 out]
              n108 = Get Date/Time String(seconds (now)=w247) -> (date string=w249:string)  [unwired: 2 in, 1 out]
              n109 = call "DateString-Days.vi"("First date"=w248, "Second date"=w249) -> ("Elapsed days"=w246:i32)  [unwired: 8 in, 1 out]
            }
            frame 5 {
              n110 = Unbundle By Name(w257) -> ("Gas Meter"=w253:timestamp)
              n111 = Get Date/Time In Seconds() -> (seconds since 1Jan1904=w256:timestamp)
              n112 = Get Date/Time String(seconds (now)=w256) -> (date string=w254:string)  [unwired: 2 in, 1 out]
              n113 = Get Date/Time String(seconds (now)=w253) -> (date string=w255:string)  [unwired: 2 in, 1 out]
              n114 = call "DateString-Days.vi"("First date"=w254, "Second date"=w255) -> ("Elapsed days"=w252:i32)  [unwired: 8 in, 1 out]
            }
            frame 6 {
              n115 = Unbundle By Name(w263) -> ("Gas Meter Pressure Transducer"=w259:timestamp)
              n116 = Get Date/Time In Seconds() -> (seconds since 1Jan1904=w262:timestamp)
              n117 = Get Date/Time String(seconds (now)=w262) -> (date string=w260:string)  [unwired: 2 in, 1 out]
              n118 = Get Date/Time String(seconds (now)=w259) -> (date string=w261:string)  [unwired: 2 in, 1 out]
              n119 = call "DateString-Days.vi"("First date"=w260, "Second date"=w261) -> ("Elapsed days"=w258:i32)  [unwired: 8 in, 1 out]
            }
            frame 7 {
              n120 = Unbundle By Name(w269) -> ("Gas Meter Thermocouple"=w265:timestamp)
              n121 = Get Date/Time In Seconds() -> (seconds since 1Jan1904=w268:timestamp)
              n122 = Get Date/Time String(seconds (now)=w268) -> (date string=w266:string)  [unwired: 2 in, 1 out]
              n123 = Get Date/Time String(seconds (now)=w265) -> (date string=w267:string)  [unwired: 2 in, 1 out]
              n124 = call "DateString-Days.vi"("First date"=w266, "Second date"=w267) -> ("Elapsed days"=w264:i32)  [unwired: 8 in, 1 out]
            }
            frame 8 {
              n125 = Get Date/Time In Seconds() -> (seconds since 1Jan1904=w274:timestamp)
              n126 = Get Date/Time String(seconds (now)=w274) -> (date string=w272:string)  [unwired: 2 in, 1 out]
              n127 = Unbundle By Name(w275) -> ("NI DAQ Card 1"=w271:timestamp)
              n128 = Get Date/Time String(seconds (now)=w271) -> (date string=w273:string)  [unwired: 2 in, 1 out]
              n129 = call "DateString-Days.vi"("First date"=w272, "Second date"=w273) -> ("Elapsed days"=w270:i32)  [unwired: 8 in, 1 out]
            }
            frame 9 {
              n130 = Get Date/Time In Seconds() -> (seconds since 1Jan1904=w280:timestamp)
              n131 = Unbundle By Name(w281) -> ("NI DAQ Card 2"=w277:timestamp)
              n132 = Get Date/Time String(seconds (now)=w280) -> (date string=w278:string)  [unwired: 2 in, 1 out]
              n133 = Get Date/Time String(seconds (now)=w277) -> (date string=w279:string)  [unwired: 2 in, 1 out]
              n134 = call "DateString-Days.vi"("First date"=w278, "Second date"=w279) -> ("Elapsed days"=w276:i32)  [unwired: 8 in, 1 out]
            }
            frame 10 {
              n135 = Get Date/Time In Seconds() -> (seconds since 1Jan1904=w286:timestamp)
              n136 = Unbundle By Name(w287) -> ("NI DAQ Card 3"=w283:timestamp)
              n137 = Get Date/Time String(seconds (now)=w286) -> (date string=w284:string)  [unwired: 2 in, 1 out]
              n138 = Get Date/Time String(seconds (now)=w283) -> (date string=w285:string)  [unwired: 2 in, 1 out]
              n139 = call "DateString-Days.vi"("First date"=w284, "Second date"=w285) -> ("Elapsed days"=w282:i32)  [unwired: 8 in, 1 out]
            }
            frame 11 {
              n140 = Get Date/Time In Seconds() -> (seconds since 1Jan1904=w292:timestamp)
              n141 = Unbundle By Name(w293) -> ("NI DAQ Card 4"=w289:timestamp)
              n142 = Get Date/Time String(seconds (now)=w292) -> (date string=w290:string)  [unwired: 2 in, 1 out]
              n143 = Get Date/Time String(seconds (now)=w289) -> (date string=w291:string)  [unwired: 2 in, 1 out]
              n144 = call "DateString-Days.vi"("First date"=w290, "Second date"=w291) -> ("Elapsed days"=w288:i32)  [unwired: 8 in, 1 out]
            }
            frame 12 {
              n145 = Get Date/Time In Seconds() -> (seconds since 1Jan1904=w298:timestamp)
              n146 = Unbundle By Name(w299) -> ("NI DAQ Card 5"=w295:timestamp)
              n147 = Get Date/Time String(seconds (now)=w298) -> (date string=w296:string)  [unwired: 2 in, 1 out]
              n148 = Get Date/Time String(seconds (now)=w295) -> (date string=w297:string)  [unwired: 2 in, 1 out]
              n149 = call "DateString-Days.vi"("First date"=w296, "Second date"=w297) -> ("Elapsed days"=w294:i32)  [unwired: 8 in, 1 out]
            }
            frame 13 {
              n150 = Get Date/Time In Seconds() -> (seconds since 1Jan1904=w304:timestamp)
              n151 = Unbundle By Name(w305) -> ("NI DAQ Card 6"=w301:timestamp)
              n152 = Get Date/Time String(seconds (now)=w304) -> (date string=w302:string)  [unwired: 2 in, 1 out]
              n153 = Get Date/Time String(seconds (now)=w301) -> (date string=w303:string)  [unwired: 2 in, 1 out]
              n154 = call "DateString-Days.vi"("First date"=w302, "Second date"=w303) -> ("Elapsed days"=w300:i32)  [unwired: 8 in, 1 out]
            }
            frame 14 {
              n155 = Get Date/Time In Seconds() -> (seconds since 1Jan1904=w310:timestamp)
              n156 = Unbundle By Name(w311) -> ("NI DAQ Card 7"=w307:timestamp)
              n157 = Get Date/Time String(seconds (now)=w310) -> (date string=w308:string)  [unwired: 2 in, 1 out]
              n158 = Get Date/Time String(seconds (now)=w307) -> (date string=w309:string)  [unwired: 2 in, 1 out]
              n159 = call "DateString-Days.vi"("First date"=w308, "Second date"=w309) -> ("Elapsed days"=w306:i32)  [unwired: 8 in, 1 out]
            }
            frame 15 {
              n160 = Get Date/Time In Seconds() -> (seconds since 1Jan1904=w316:timestamp)
              n161 = Unbundle By Name(w317) -> ("TC Panel 1"=w313:timestamp)
              n162 = Get Date/Time String(seconds (now)=w316) -> (date string=w314:string)  [unwired: 2 in, 1 out]
              n163 = Get Date/Time String(seconds (now)=w313) -> (date string=w315:string)  [unwired: 2 in, 1 out]
              n164 = call "DateString-Days.vi"("First date"=w314, "Second date"=w315) -> ("Elapsed days"=w312:i32)  [unwired: 8 in, 1 out]
            }
            frame 16 {
              n165 = Unbundle By Name(w323) -> ("TC Panel 2"=w319:timestamp)
              n166 = Get Date/Time In Seconds() -> (seconds since 1Jan1904=w322:timestamp)
              n167 = Get Date/Time String(seconds (now)=w322) -> (date string=w320:string)  [unwired: 2 in, 1 out]
              n168 = Get Date/Time String(seconds (now)=w319) -> (date string=w321:string)  [unwired: 2 in, 1 out]
              n169 = call "DateString-Days.vi"("First date"=w320, "Second date"=w321) -> ("Elapsed days"=w318:i32)  [unwired: 8 in, 1 out]
            }
            frame 17 {
              n170 = Unbundle By Name(w329) -> ("Probe 1 Temp"=w325:timestamp)
              n171 = Get Date/Time In Seconds() -> (seconds since 1Jan1904=w328:timestamp)
              n172 = Get Date/Time String(seconds (now)=w328) -> (date string=w326:string)  [unwired: 2 in, 1 out]
              n173 = Get Date/Time String(seconds (now)=w325) -> (date string=w327:string)  [unwired: 2 in, 1 out]
              n174 = call "DateString-Days.vi"("First date"=w326, "Second date"=w327) -> ("Elapsed days"=w324:i32)  [unwired: 8 in, 1 out]
            }
            frame 18 {
              n175 = Unbundle By Name(w335) -> ("Probe 2 Temp"=w331:timestamp)
              n176 = Get Date/Time In Seconds() -> (seconds since 1Jan1904=w334:timestamp)
              n177 = Get Date/Time String(seconds (now)=w334) -> (date string=w332:string)  [unwired: 2 in, 1 out]
              n178 = Get Date/Time String(seconds (now)=w331) -> (date string=w333:string)  [unwired: 2 in, 1 out]
              n179 = call "DateString-Days.vi"("First date"=w332, "Second date"=w333) -> ("Elapsed days"=w330:i32)  [unwired: 8 in, 1 out]
            }
            frame 19 {
              n180 = Unbundle By Name(w341) -> ("Chamber Temp"=w337:timestamp)
              n181 = Get Date/Time In Seconds() -> (seconds since 1Jan1904=w340:timestamp)
              n182 = Get Date/Time String(seconds (now)=w340) -> (date string=w338:string)  [unwired: 2 in, 1 out]
              n183 = Get Date/Time String(seconds (now)=w337) -> (date string=w339:string)  [unwired: 2 in, 1 out]
              n184 = call "DateString-Days.vi"("First date"=w338, "Second date"=w339) -> ("Elapsed days"=w336:i32)  [unwired: 8 in, 1 out]
            }
          }
        }
        n185 = Array Max & Min(array=w207) -> (min value=w204:i32)  [unwired: 3 out]
        n186 = Less?(x=w204, y=30) -> (x < y?=w205:bool)
        n187 = Number To Decimal String(number=w204) -> (decimal integer string=w203:string)  [unwired: 1 in]
        n188 = case shown="True" w205 {
          tunnel: w203 -> [_ w217]
          frame False {
          }
          frame True {
            n189 = Concatenate Strings("Componets will be out of calibration in " ("message"), w217, " Days" ("string")) -> (w214:string)
            n190 = One Button Dialog(message=w214, button name ("OK")="OK") -> ()  [unwired: 1 out]
          }
        }
        n191 = call <vilib>:"Add State(s) to Queue__jki_lib_state_machine.vi"("State(s) in (\"\")"=w213) -> ("States Out"=w212:string)  [unwired: 14 in]
      }
      frame "Write Calibration Date" {
        # "Your code here.\n(You can make a copy of, or modify, this frame)"
        n192 = Unbundle By Name(w348) -> ("Calibration\nDue Date"=w349:T3, "Total Array"=w344:string[][])  [unwired: 1 out]
        n193 = for {
          N: 20 -> [_]
          tunnel: w349 -> [w363]
          tunnel: string[] [] -> [w361]
          tunnel: [w360] -> w346 mode=indexing
          tunnel: [w356] -> w350
          tunnel: w351 -> [w356]
          i -> [w362]
          n194 = case shown="15" w362 {
            tunnel: w363 -> [w366 w369 w372 w375 w378 w381 w384 w387 w390 w393 w396 w399 w402 w405 w408 w411 w414 w417 w419 w423]
            tunnel: [w364 w367 w370 w373 w376 w379 w382 w385 w388 w391 w394 w397 w400 w403 w406 w409 w412 w415 w420 w421] -> w359
            frame 0, Default {
              n195 = Unbundle By Name(w366) -> ("Chroma"=w365:timestamp)
              n196 = Format Date/Time String(seconds (now)=w365) -> (date/time string=w364:string)  [unwired: 2 in]
            }
            frame 1 {
              n197 = Unbundle By Name(w369) -> ("WT 500"=w368:timestamp)
              n198 = Format Date/Time String(seconds (now)=w368) -> (date/time string=w367:string)  [unwired: 2 in]
            }
            frame 2 {
              n199 = Unbundle By Name(w372) -> ("Barometer"=w371:timestamp)
              n200 = Format Date/Time String(seconds (now)=w371) -> (date/time string=w370:string)  [unwired: 2 in]
            }
            frame 3 {
              n201 = Unbundle By Name(w375) -> ("B-Tech Scale"=w374:timestamp)
              n202 = Format Date/Time String(seconds (now)=w374) -> (date/time string=w373:string)  [unwired: 2 in]
            }
            frame 4 {
              n203 = Unbundle By Name(w378) -> ("Sentra Scale"=w377:timestamp)
              n204 = Format Date/Time String(seconds (now)=w377) -> (date/time string=w376:string)  [unwired: 2 in]
            }
            frame 5 {
              n205 = Unbundle By Name(w381) -> ("Gas Meter"=w380:timestamp)
              n206 = Format Date/Time String(seconds (now)=w380) -> (date/time string=w379:string)  [unwired: 2 in]
            }
            frame 6 {
              n207 = Unbundle By Name(w384) -> ("Gas Meter Pressure Transducer"=w383:timestamp)
              n208 = Format Date/Time String(seconds (now)=w383) -> (date/time string=w382:string)  [unwired: 2 in]
            }
            frame 7 {
              n209 = Unbundle By Name(w387) -> ("Gas Meter Thermocouple"=w386:timestamp)
              n210 = Format Date/Time String(seconds (now)=w386) -> (date/time string=w385:string)  [unwired: 2 in]
            }
            frame 8 {
              n211 = Unbundle By Name(w390) -> ("NI DAQ Card 1"=w389:timestamp)
              n212 = Format Date/Time String(seconds (now)=w389) -> (date/time string=w388:string)  [unwired: 2 in]
            }
            frame 9 {
              n213 = Unbundle By Name(w393) -> ("NI DAQ Card 2"=w392:timestamp)
              n214 = Format Date/Time String(seconds (now)=w392) -> (date/time string=w391:string)  [unwired: 2 in]
            }
            frame 10 {
              n215 = Unbundle By Name(w396) -> ("NI DAQ Card 3"=w395:timestamp)
              n216 = Format Date/Time String(seconds (now)=w395) -> (date/time string=w394:string)  [unwired: 2 in]
            }
            frame 11 {
              n217 = Unbundle By Name(w399) -> ("NI DAQ Card 4"=w398:timestamp)
              n218 = Format Date/Time String(seconds (now)=w398) -> (date/time string=w397:string)  [unwired: 2 in]
            }
            frame 12 {
              n219 = Unbundle By Name(w402) -> ("NI DAQ Card 5"=w401:timestamp)
              n220 = Format Date/Time String(seconds (now)=w401) -> (date/time string=w400:string)  [unwired: 2 in]
            }
            frame 13 {
              n221 = Unbundle By Name(w405) -> ("NI DAQ Card 6"=w404:timestamp)
              n222 = Format Date/Time String(seconds (now)=w404) -> (date/time string=w403:string)  [unwired: 2 in]
            }
            frame 14 {
              n223 = Unbundle By Name(w408) -> ("NI DAQ Card 7"=w407:timestamp)
              n224 = Format Date/Time String(seconds (now)=w407) -> (date/time string=w406:string)  [unwired: 2 in]
            }
            frame 15 {
              n225 = Unbundle By Name(w411) -> ("TC Panel 1"=w410:timestamp)
              n226 = Format Date/Time String(seconds (now)=w410) -> (date/time string=w409:string)  [unwired: 2 in]
            }
            frame 16 {
              n227 = Unbundle By Name(w414) -> ("TC Panel 2"=w413:timestamp)
              n228 = Format Date/Time String(seconds (now)=w413) -> (date/time string=w412:string)  [unwired: 2 in]
            }
            frame 17 {
              n229 = Unbundle By Name(w417) -> ("Probe 1 Temp"=w416:timestamp)
              n230 = Format Date/Time String(seconds (now)=w416) -> (date/time string=w415:string)  [unwired: 2 in]
            }
            frame 18 {
              n231 = Unbundle By Name(w419) -> ("Probe 2 Temp"=w418:timestamp)
              n232 = Format Date/Time String(seconds (now)=w418) -> (date/time string=w420:string)  [unwired: 2 in]
            }
            frame 19 {
              n233 = Unbundle By Name(w423) -> ("Chamber Temp"=w422:timestamp)
              n234 = Format Date/Time String(seconds (now)=w422) -> (date/time string=w421:string)  [unwired: 2 in]
            }
          }
          n235 = call <vilib>:"Space Constant.vi"() -> ("String"=w357:string)
          n236 = Match Pattern(string=w359, regular expression=w357) -> (before substring=w358:string)  [unwired: 1 in, 3 out]
          n237 = Build Array (concatenate)(w361, w358) -> (w360:string[])
        }
        n238 = call "Array-Get 1D str Column fr 2D.vi"("2D Array Data"=w346, "column index"=0) -> ("Column Data"=w343:string[])  [unwired: 13 in]
        n239 = Build Array (concatenate)(w344, w343) -> (w342:string[][])
        n240 = Bundle By Name(cluster=w348, "Total Array"=w342) -> (w347:T6)
        n241 = call <vilib>:"Add State(s) to Queue__jki_lib_state_machine.vi"("State(s) in (\"\")"=w355) -> ("States Out"=w354:string)  [unwired: 14 in]
      }
      frame "Write to File" {
        # "Your code here.\n(You can make a copy of, or modify, this frame)"
        n242 = Unbundle By Name(w431) -> ("file path (dialog if empty)"=w430:path, "Total Array"=w426:string[][])
        n243 = Build Array (concatenate)(string[] ["Chroma", "WT 500", "Barometer", "B-Tech Scale", "Sentra Scale", "Gas Meter", "Gas Meter Pressure Transducer", "Gas Meter Thermocouple", "NI DAQ Card 1", "NI DAQ Card 2", "NI DAQ Card 3", "NI DAQ Card 4", "NI DAQ Card 5", "NI DAQ Card 6", "NI DAQ Card 7", "TC Panel 1", "TC Panel 2", "Probe 1 Temp", "Probe 2 Temp", "Chamber Temp"], w426) -> (w425:string[][])
        n244 = Transpose 2D Array(2D array=w425) -> (transposed array=w424:string[][])
        "OutputData" <- w424
        n245 = call-poly <vilib>:"Write To Spreadsheet File.vi"("delimiter (\\t)"="," ("delimiter (\\t)"), "2D data"=w424, "file path (dialog if empty)"=w430) -> ()  [unwired: 5 in, 1 out]
        n246 = call <vilib>:"Add State(s) to Queue__jki_lib_state_machine.vi"("State(s) in (\"\")"=w433) -> ("States Out"=w432:string)  [unwired: 14 in]
      }
      frame "Write Calibration ID" {
        # "Your code here.\n(You can make a copy of, or modify, this frame)"
        n247 = Unbundle By Name(w441) -> ("Calibration ID"=w439:T2, "Total Array"=w438:string[][])
        n248 = for {
          N: 20 -> [_]
          tunnel: w439 -> [w453]
          tunnel: string[] [] -> [w451]
          tunnel: [w450] -> w436 mode=indexing
          tunnel: [w449] -> w442
          tunnel: w443 -> [w449]
          i -> [w452]
          n249 = case shown="15" w452 {
            tunnel: w453 -> [w455 w457 w459 w461 w463 w465 w467 w469 w471 w473 w475 w477 w479 w481 w483 w485 w487 w488 w491 w493]
            tunnel: [w454 w456 w458 w460 w462 w464 w466 w468 w470 w472 w474 w476 w478 w480 w482 w484 w486 w489 w490 w492] -> w448
            frame 0, Default {
              n250 = Unbundle By Name(w455) -> ("Chroma"=w454:string)
            }
            frame 1 {
              n251 = Unbundle By Name(w457) -> ("WT 500"=w456:string)
            }
            frame 2 {
              n252 = Unbundle By Name(w459) -> ("Barometer"=w458:string)
            }
            frame 3 {
              n253 = Unbundle By Name(w461) -> ("B-Tech Scale"=w460:string)
            }
            frame 4 {
              n254 = Unbundle By Name(w463) -> ("Sentra Scale"=w462:string)
            }
            frame 5 {
              n255 = Unbundle By Name(w465) -> ("Gas Meter"=w464:string)
            }
            frame 6 {
              n256 = Unbundle By Name(w467) -> ("Gas Meter Pressure Transducer"=w466:string)
            }
            frame 7 {
              n257 = Unbundle By Name(w469) -> ("Gas Meter Thermocouple"=w468:string)
            }
            frame 8 {
              n258 = Unbundle By Name(w471) -> ("NI DAQ Card 1"=w470:string)
            }
            frame 9 {
              n259 = Unbundle By Name(w473) -> ("NI DAQ Card 2"=w472:string)
            }
            frame 10 {
              n260 = Unbundle By Name(w475) -> ("NI DAQ Card 3"=w474:string)
            }
            frame 11 {
              n261 = Unbundle By Name(w477) -> ("NI DAQ Card 4"=w476:string)
            }
            frame 12 {
              n262 = Unbundle By Name(w479) -> ("NI DAQ Card 5"=w478:string)
            }
            frame 13 {
              n263 = Unbundle By Name(w481) -> ("NI DAQ Card 6"=w480:string)
            }
            frame 14 {
              n264 = Unbundle By Name(w483) -> ("NI DAQ Card 7"=w482:string)
            }
            frame 15 {
              n265 = Unbundle By Name(w485) -> ("TC Panel 1"=w484:string)
            }
            frame 16 {
              n266 = Unbundle By Name(w487) -> ("TC Panel 2"=w486:string)
            }
            frame 17 {
              n267 = Unbundle By Name(w488) -> ("Probe 1 Temp"=w489:string)
            }
            frame 18 {
              n268 = Unbundle By Name(w491) -> ("Probe 2 Temp"=w490:string)
            }
            frame 19 {
              n269 = Unbundle By Name(w493) -> ("Chamber Temp"=w492:string)
            }
          }
          n270 = Build Array (concatenate)(w451, w448) -> (w450:string[])
        }
        n271 = call "Array-Get 1D str Column fr 2D.vi"("2D Array Data"=w436, "column index"=0) -> ("Column Data"=w434:string[])  [unwired: 13 in]
        n272 = Build Array (concatenate)(w438, w434) -> (w437:string[][])
        n273 = Bundle By Name(cluster=w441, "Total Array"=w437) -> (w440:T6)
        n274 = call <vilib>:"Add State(s) to Queue__jki_lib_state_machine.vi"("State(s) in (\"\")"=w447) -> ("States Out"=w446:string)  [unwired: 14 in]
      }
      frame "Write Calibration SN" {
        # "Your code here.\n(You can make a copy of, or modify, this frame)"
        n275 = Unbundle By Name(w501) -> ("SN"=w499:T1, "Total Array"=w498:string[][])
        n276 = for {
          N: 20 -> [_]
          tunnel: w499 -> [w513]
          tunnel: string[] [] -> [w511]
          tunnel: [w510] -> w496 mode=indexing
          tunnel: [w509] -> w502
          tunnel: w503 -> [w509]
          i -> [w512]
          n277 = case shown="15" w512 {
            tunnel: w513 -> [w515 w517 w519 w521 w523 w525 w527 w529 w531 w533 w535 w537 w539 w541 w543 w545 w547 w549 w551 w553]
            tunnel: [w514 w516 w518 w520 w522 w524 w526 w528 w530 w532 w534 w536 w538 w540 w542 w544 w546 w548 w550 w552] -> w508
            frame 0, Default {
              n278 = Unbundle By Name(w515) -> ("Chroma"=w514:string)
            }
            frame 1 {
              n279 = Unbundle By Name(w517) -> ("WT 500"=w516:string)
            }
            frame 2 {
              n280 = Unbundle By Name(w519) -> ("Barometer"=w518:string)
            }
            frame 3 {
              n281 = Unbundle By Name(w521) -> ("B-Tech Scale"=w520:string)
            }
            frame 4 {
              n282 = Unbundle By Name(w523) -> ("Sentra Scale"=w522:string)
            }
            frame 5 {
              n283 = Unbundle By Name(w525) -> ("Gas Meter"=w524:string)
            }
            frame 6 {
              n284 = Unbundle By Name(w527) -> ("Gas Meter Pressure Transducer"=w526:string)
            }
            frame 7 {
              n285 = Unbundle By Name(w529) -> ("Gas Meter Thermocouple"=w528:string)
            }
            frame 8 {
              n286 = Unbundle By Name(w531) -> ("NI DAQ Card 1"=w530:string)
            }
            frame 9 {
              n287 = Unbundle By Name(w533) -> ("NI DAQ Card 2"=w532:string)
            }
            frame 10 {
              n288 = Unbundle By Name(w535) -> ("NI DAQ Card 3"=w534:string)
            }
            frame 11 {
              n289 = Unbundle By Name(w537) -> ("NI DAQ Card 4"=w536:string)
            }
            frame 12 {
              n290 = Unbundle By Name(w539) -> ("NI DAQ Card 5"=w538:string)
            }
            frame 13 {
              n291 = Unbundle By Name(w541) -> ("NI DAQ Card 6"=w540:string)
            }
            frame 14 {
              n292 = Unbundle By Name(w543) -> ("NI DAQ Card 7"=w542:string)
            }
            frame 15 {
              n293 = Unbundle By Name(w545) -> ("TC Panel 1"=w544:string)
            }
            frame 16 {
              n294 = Unbundle By Name(w547) -> ("TC Panel 2"=w546:string)
            }
            frame 17 {
              n295 = Unbundle By Name(w549) -> ("Probe 1 Temp"=w548:string)
            }
            frame 18 {
              n296 = Unbundle By Name(w551) -> ("Probe 2 Temp"=w550:string)
            }
            frame 19 {
              n297 = Unbundle By Name(w553) -> ("Chamber Temp"=w552:string)
            }
          }
          n298 = Build Array (concatenate)(w511, w508) -> (w510:string[])
        }
        n299 = call "Array-Get 1D str Column fr 2D.vi"("2D Array Data"=w496, "column index"=0) -> ("Column Data"=w494:string[])  [unwired: 13 in]
        "snta" <- w494
        n300 = Build Array (concatenate)(w498, w494) -> (w497:string[][])
        n301 = Bundle By Name(cluster=w501, "Total Array"=w497) -> (w500:T6)
        n302 = call <vilib>:"Add State(s) to Queue__jki_lib_state_machine.vi"("State(s) in (\"\")"=w507) -> ("States Out"=w506:string)  [unwired: 14 in]
      }
    }
  }
  "error out" <- w2
